vi "ConvertTagReadToInfo.vi"(11 "Bytes Read":u8[](array[numeric]) format="%02x") -> (2 "UID":string, 3 "# of tags":u8)   [LabVIEW 2015]
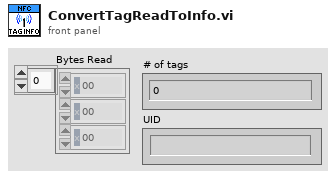
[diagram p1: front panel]
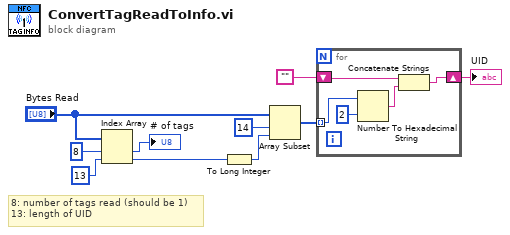
[diagram p0: block diagram]
diagram:
  # "8: number of tags read (should be 1)\n13: length of UID"
  n1 = Index Array(array="Bytes Read", index #1=8 ("index"), index #2=13 ("index")) -> (element #1=→"# of tags":u8, element #2=w6:u8)
  n2 = To Long Integer(number=w6) -> (32bit integer=w5:i32)
  n3 = Array Subset(array="Bytes Read", index=14, length=w5) -> (w3:u8[])
  n4 = for {
    tunnel: w3 -> [w15] mode=indexing
    shift-right: [w11] -> w1
    shift-left: "" -> [w13]
    n5 = Number To Hexadecimal String(1:i16 2 ("width (-)"), 2:w15) -> (0:w12:string)
    n6 = Concatenate Strings(w13, w12) -> (w11:string)
  }
  "UID" <- w1
